vi "Stop Core.vi"(10 "final error code":i32, 11 "State Actor in":refnum<class "State Actor.lvclass">) -> (3 "State Actor out":refnum<class "State Actor.lvclass">)   [LabVIEW 2024, in "State Actor.lvlib" / "State Actor.lvclass"]
doc: "<p>(<strong>Filename</strong>: <span class=\"dnl\">Actor Framework.lvlib:Actor.lvclass:Stop Core.vi</span>)</p>\n<p>Defines what the actor does before it stops. Use the <strong>final error code</strong> input to determine whether the actor shut down in response to an error.</p>\n<p>By default, this method passes the Stop message along to all <a href=\"nihelplauncher://docs/csh?context=lvcore_lvcomm_af_launch_nested_actor\">auto-stop nested actors</a>. A descendant class may override this method to define additional behavior, such as shutting down any processes the actor initiated in its override of the <a href=\"nihelplauncher://docs/csh?context=lvcore_lvcomm_af_actor_core\">Actor Core</a> method.</p>"
uses:
  State Actor.lvclass
  State Actor.lvclass/State Actor.ctl
  <vilib>/ActorFramework/Actor/Actor.lvclass
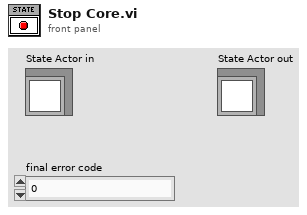
[diagram p1: front panel]
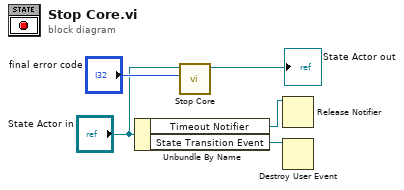
[diagram p0: block diagram]
diagram:
  n1 = Unbundle By Name("State Actor in") -> ("Timeout Notifier"=w2:refnum<notifier>, "State Transition Event"=w1:refnum<user-event>)
  n2 = call-parent "Stop Core.vi"("final error code"="final error code", "Actor in"="State Actor in") -> ("Actor out"=→"State Actor out":refnum<class "State Actor.lvclass">)  [unwired: 9 in]
  n3 = Release Notifier(notifier=w2) -> ()  [unwired: 2 in, 3 out]
  n4 = Destroy User Event(user event=w1) -> ()  [unwired: 1 in, 1 out]
